vi "HandleExit.vi"(8 "error in (no error)":errorcluster, 9 "VI Refnum":refnum<vi>, 10 "StopArgument":variant, 11 "ModuleAdmin":refnum<class "ModuleAdmin.lvclass">) -> (0 "error out":errorcluster, 1 "Exit via Stop Module Req?":bool, 2 "WaitForStop?":bool)   [LabVIEW 2018, in "ScopePlugins.lvlib"]
uses:
  ScopePlugins/ScopePlugins.lvlib
  <userlib>/NIST/ModuleAdminLib/ModuleAdmin/ModuleAdmin.lvclass
  C:/Program Files (x86)/National Instruments/LabVIEW 2018/user.lib/NIST/ModuleAdminLib/ModuleAdminBase/ModuleAdminBase.lvclass
  PublicAPI/Arguments/Requests/clStopArgument.ctl
  ScopeShared/ScopeShared.lvlib
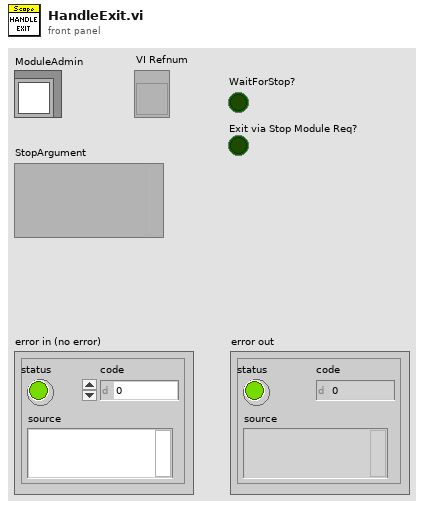
[diagram p1: front panel]
types:
  T1 = typedef "ScopeShared.lvlib/clStopArgument.ctl" = cluster{"Exit via Stop Module Req?":bool, "Wait for Module to stop?":bool, "ModuleAdmin":refnum<class "ModuleAdmin.lvclass">}
  T2 = enum32{"Invalid", "Standard", "Closed", "Hidden", "Minimized", "Maximized"}
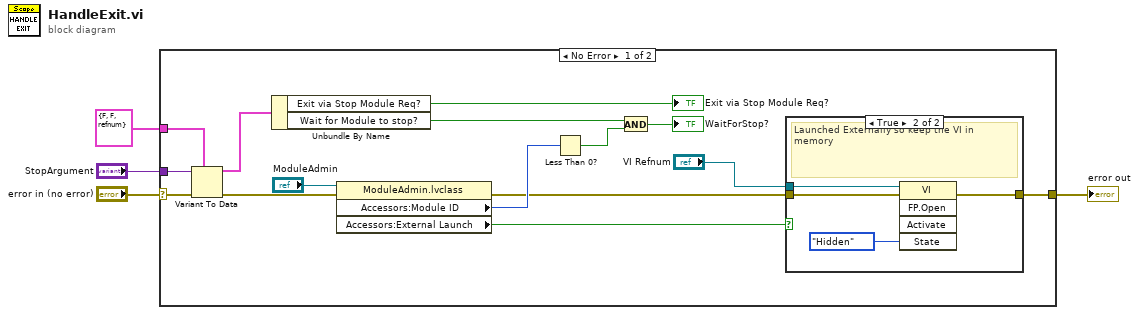
[diagram p0: block diagram]
diagram:
  n1 = case shown="No Error" "error in (no error)" {
    selector: "error in (no error)" -> [w7 w25]
    tunnel: [w17 w25] -> w4
    tunnel: T1 {"Exit via Stop Module Req?"=FALSE, "Wait for Module to stop?"=FALSE, "ModuleAdmin"=refnum} ("Stop Argument") -> [w16 _]
    tunnel: "StopArgument" -> [w14 _]
    frame No Error {
      n2 = Variant To Data(error in=w7, type=w16, Variant=w14) -> (data=w15:T1, error out=w6:errorcluster)
      n3 = Unbundle By Name(w15) -> ("Exit via Stop Module Req?"=→"Exit via Stop Module Req?":bool, "Wait for Module to stop?"=w10:bool)
      n4 = property class="ModuleAdmin.lvclass"(reference="ModuleAdmin", error in=w6) -> (error out=w5:errorcluster, "Accessors:Module ID"=w11:i32, "Accessors:External Launch"=w13:bool)  [unwired: 1 out]
      n5 = Less Than 0?(x=w11) -> (x < 0?=w19:bool)
      n6 = And(x=w10, y=w19) -> (x .and. y?=→"WaitForStop?":bool)
      n7 = case shown="True" w13 {
        tunnel: "VI Refnum" -> [_ w24]
        tunnel: [w20 w22] -> w17
        tunnel: w5 -> [w20 w21]
        frame False {
        }
        frame True {
          # "Launched Externally so keep the VI in memory"
          n8 = invoke class="VI" method="FP.Open"(reference=w24, error in=w21, "State"=T2."Hidden") -> (error out=w22:errorcluster)  [unwired: 2 in, 4 out]
        }
      }
    }
    frame Error {
    }
  }
  "error out" <- w4
